vi "Name.vi"(1 "Hash Function in":refnum<class "NI_SHA-256.lvclass">) -> (0 "String":string)   [LabVIEW 2013, in "NI_SHA-256(2013).lvlib" / "NI_SHA-256.lvclass"]
uses:
  NI_SHA-256.lvclass
  NI_SHA-256.lvclass/NI_SHA-256.ctl
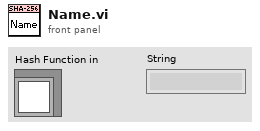
[diagram p1: front panel]
types:
  T1 = typedef "NI_SHA-256(2013).lvlib/NI_SHA-256.lvclass/Mode.ctl" = enum16{"SHA-256", "SHA-224"}
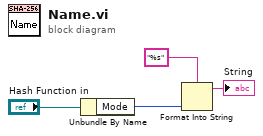
[diagram p0: block diagram]
diagram:
  n1 = Unbundle By Name("Hash Function in") -> ("Mode"=w2:T1)
  n2 = Format Into String(format string="%s", w2) -> (resulting string=→"String":string)  [unwired: 2 in, 1 out]
